vi "test VI.vi"(8 "error in (no error)":errorcluster, 9 "Array":T2[](array[typedef]) format="%.0x", 10 "Device Item Ref":T2 format="%.0x", 11 "Boolean":bool) -> (0 "error out":errorcluster)   [LabVIEW 2009, in "PXI-4130 Custom Device.lvlib"]
uses:
  PXI-4130 Custom Device.lvlib
  <vilib>/NI VeriStand/Custom Device API/Custom Device Item Ref.ctl
  <vilib>/NI VeriStand/Custom Device API/Custom Device Item Info.ctl
  <vilib>/NI VeriStand/Custom Device API/Custom Device API.lvlib
panel:
  in  "OK Button":bool
  out "Array 3":bool[](array[boolean])
  out "Found":bool
  out "Array 2":T1[](array[typedef])
  out "Item Info":T1
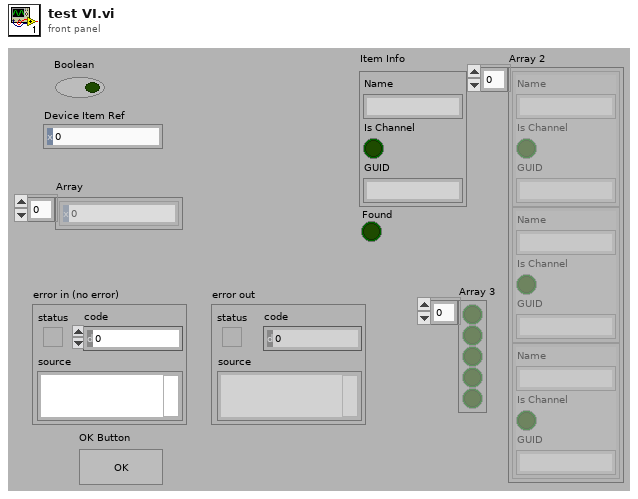
[diagram p1: front panel]
types:
  T1 = typedef "Custom Device API.lvlib/Custom Device Item Info.ctl" = cluster{"Name":string, "Is Channel":bool, "GUID":string}
  T2 = typedef "Custom Device API.lvlib/Custom Device Item Ref.ctl" = u64
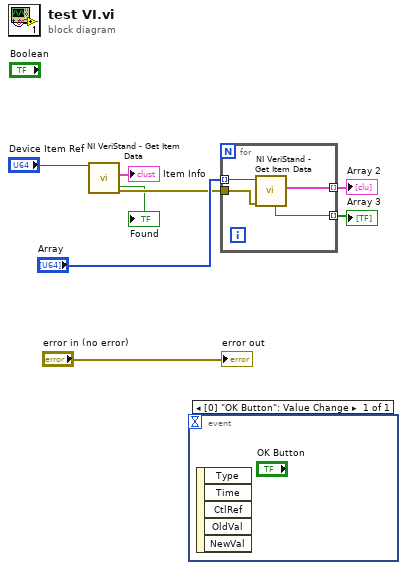
[diagram p0: block diagram]
diagram:
  n1 = call <vilib>:"NI VeriStand - Get Item Data.vi"("Item Ref in"="Device Item Ref") -> ("error out"=w5:errorcluster, "Item Info"=→"Item Info":T1, "Found"=→"Found":bool)  [unwired: 7 in, 1 out]
  n2 = event shown="[0] \"OK Button\": Value Change" {
    selector: _ -> [_]
    dyn-events: _ -> [_]
    timeout: _ -> [_]
    event [0] "OK Button": Value Change {
      n3 = event-data() -> ()  [unwired: 1 in, 5 out]
    }
  }
  n4 = for {
    tunnel: "Array" -> [w12] mode=indexing
    tunnel: w5 -> [w11]
    tunnel: [w10] -> w4 mode=indexing
    tunnel: [w9] -> w2 mode=indexing
    n5 = call <vilib>:"NI VeriStand - Get Item Data.vi"("error in (no error)"=w11, "Item Ref in"=w12) -> ("Item Info"=w10:T1, "Found"=w9:bool)  [unwired: 6 in, 2 out]
  }
  "Array 2" <- w4
  "Array 3" <- w2
  "error out" <- "error in (no error)"
